vi "Metronome-FINAL.vi"() -> ()   [LabVIEW 2014]
panel:
  in  "stop":bool
  in  "Beats Per Minute":dbl
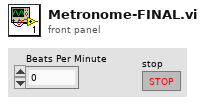
[diagram p1: front panel]
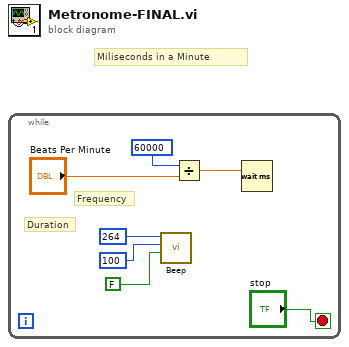
[diagram p0: block diagram]
diagram:
  # "Miliseconds in a Minute"
  n1 = while {
    stop <- "stop" stop-if-true
    # "Duration"
    # "Frequency"
    n2 = call <vilib>:"Beep.vi"("use system alert? (T) - ignored"=FALSE ("use system alert? (T)"), "duration (msec) - ignored"=u32 100 ("duration (msec)"), "frequency (Hz) - ignored"=u32 264 ("frequency (Hz)")) -> ()  [unwired: 9 in]
    n3 = Divide(x=60000, y="Beats Per Minute") -> (x/y=w5:dbl)
    n4 = Wait (ms)(milliseconds to wait=w5) -> ()  [unwired: 1 out]
  }
